vi "Close Sessions DC Power.vi"(11 "Semiconductor Module Context":T1) -> (0 "error out":errorcluster)   [LabVIEW 2013]
uses:
  <vilib>/NI_TestStand_SemiconductorModule/NI_TestStand_Semiconductor_Module.lvlibp/PinMap/General/SemiconductorModuleContext.ctl
  <vilib>/NI_TestStand_SemiconductorModule/NI_TestStand_Semiconductor_Module.lvlibp
panel:
  out "Instrument Sessions":refnum<k15>[](array[refnum])
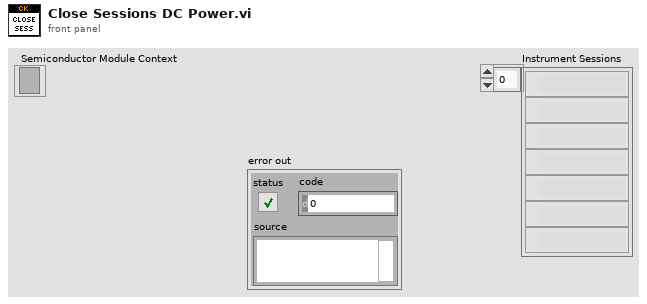
[diagram p1: front panel]
types:
  T1 = typedef "NI_TestStand_Semiconductor_Module.lvlibp/SemiconductorModuleContext.ctl" = refnum<k7>
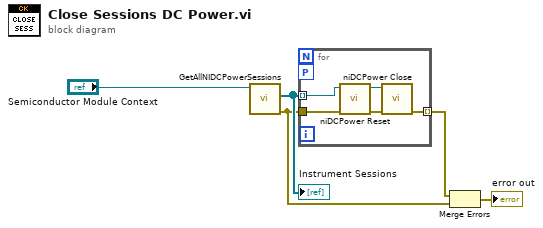
[diagram p0: block diagram]
diagram:
  n1 = call <vilib>:"GetAllNIDCPowerSessions.vi"("Semiconductor Module Context"="Semiconductor Module Context") -> ("error out"=w2:errorcluster, "Instrument Sessions"=w5:refnum<k15>[])  [unwired: 8 in, 1 out]
  "Instrument Sessions" <- w5
  n2 = for {
    tunnel: w2 -> [w9]
    tunnel: w5 -> [w8] mode=indexing
    tunnel: [w10] -> w3 mode=indexing
    workers-P: _ -> [_]
    n3 = call <instrlib>:"niDCPower Reset.vi"("error in (no error)"=w9, "instrument handle"=w8) -> ("error out"=w6:errorcluster, "instrument handle out"=w7:refnum<k15>)  [unwired: 8 in]
    n4 = call <instrlib>:"niDCPower Close.vi"("error in (no error)"=w6, "instrument handle"=w7) -> ("error out"=w10:errorcluster)  [unwired: 9 in]
  }
  n5 = Merge Errors(w3, w2) -> (→"error out":errorcluster)
